vi "PicoScope4000aExampleRapidBlock.vi"() -> ()   [LabVIEW 2016]
uses:
  PicoScope4000aLib/PicoScope4000aAnalogChannelSettings.ctl
panel:
  out "USB 3.0 on non-USB 3.0 port":bool=TRUE
  out "USB powered":bool=TRUE
  in  "Trigger Settings":T1={"Trigger Enabled"=FALSE, "Trigger Source"=enum."Channel A", "Trigger Threshold (Volts/Probe Units)"=0.0, "Trigger Direction"=2, "Trigger Delay (samples)"=0, "Auto Trigger Time (ms)"=0} {"Trigger Direction" items=["Rising"=2, "Falling"=3]}
  in  "Resolution":u32(ring)=1 items=["8-bit", "12-bit", "14-bit"]
  in  "Serial Number":string
  in  "Open using Serial Number":bool
  in  "Channel A Settings":T2={"Enabled"=TRUE, "Coupling"=1, "Range"=6, "Analogue Offset"=0.0, "Bandwidth Limit"=0} {"Bandwidth Limit" items=["Full", "20kHz", "100kHz", "1MHz"]; "Range" items=["10 mV", "20 mV", "50 mV", "100 mV", "200 mV", "500 mV", "1 V", "2 V", "5 V", "10 V", "20 V", "50 V ", "100 V"]; "Coupling" items=["AC", "DC"]}
  in  "Rapid Block Acquisition Settings":T3={"preTriggerSamples"=0, "postTriggerSamples"=1024, "timebase"=10, "Number of Captures"=100}
  out "Capture Complete":bool
  in  "Run":bool
  out "Channel A":i16[][](graph)
  in  "Capture Index":i16 min=0
  in  "stop":bool
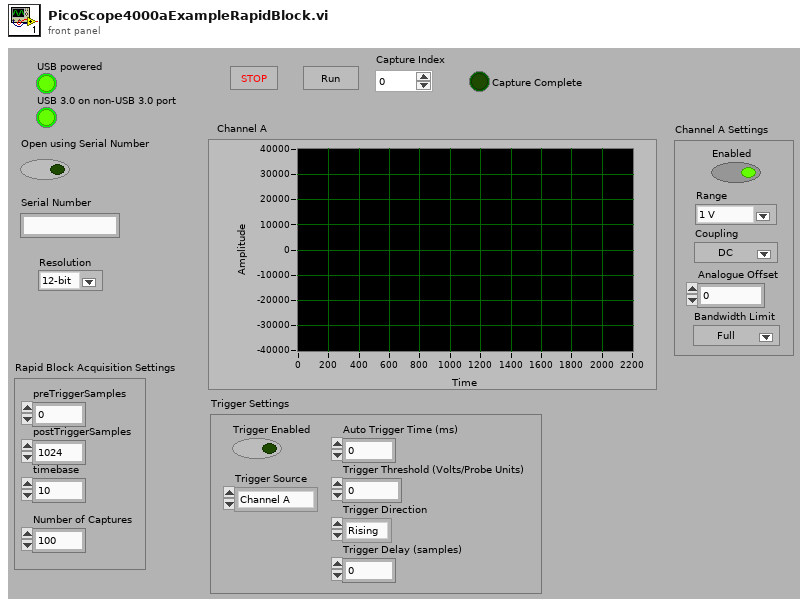
[diagram p1: front panel]
types:
  T1 = cluster{"Trigger Enabled":bool, "Trigger Source":enum16{"Channel A", "Channel B", "Channel C", "Channel D", "Channel E", "Channel F", "Channel G", "Channel H"}, "Trigger Threshold (Volts/Probe Units)":dbl, "Trigger Direction":u16, "Trigger Delay (samples)":u32, "Auto Trigger Time (ms)":i16}
  T2 = typedef "PicoScope4000aAnalogChannelSettings.ctl" = cluster{"Enabled":bool, "Coupling":i16, "Range":u16, "Analogue Offset":sgl, "Bandwidth Limit":u32}
  T3 = cluster{"preTriggerSamples":u32, "postTriggerSamples":u32, "timebase":u32, "Number of Captures":u32}
  T4 = cluster{"Driver Version":string, "USB Version":string, "Hardware":string, "Variant":string, "Batch and Serial":string, "Cal Date":string, "Kernel Version":string, "Digital HW Version":string, "Analogue HW Version":string, "Firmware 1":string, "Firmware 2":string, "Num. channels":i16}
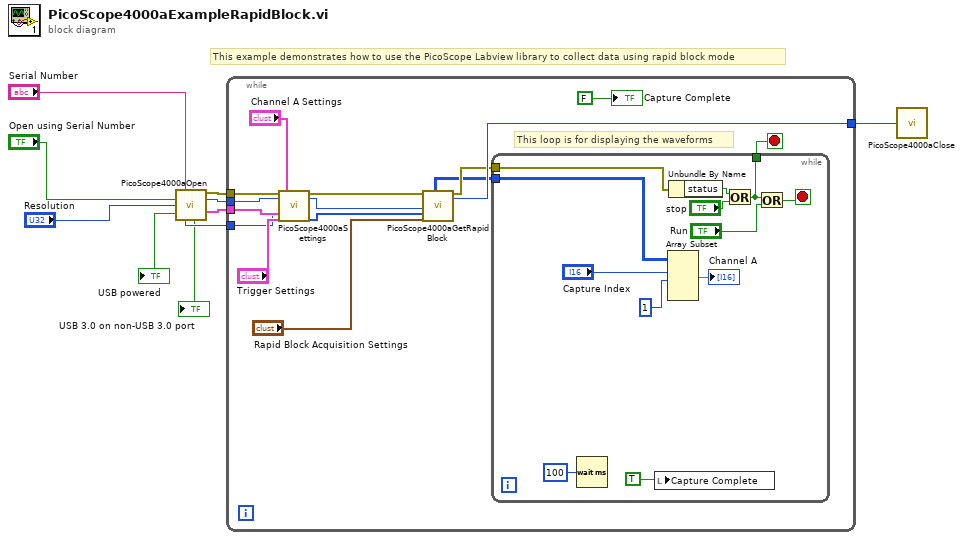
[diagram p0: block diagram]
diagram:
  # "This example demonstrates how to use the PicoScope Labview library to collect data using rapid block mode"
  n1 = call "PicoScope4000aOpen.vi"("Serial Number"="Serial Number", "Use Serial Number"="Open using Serial Number", "Resolution"="Resolution") -> ("error out"=w7:errorcluster, "handle"=w6:i16, "Unit Info"=w5:T4, "Max ADC value"=w3:i16, "USB powered"=→"USB powered":bool, "USB 3.0 on non-USB 3.0 port"=→"USB 3.0 on non-USB 3.0 port":bool)  [unwired: 7 in]
  n2 = while {
    tunnel: [w17] -> w10
    tunnel: w7 -> [w22]
    tunnel: w6 -> [w23]
    tunnel: w5 -> [w13]
    tunnel: w3 -> [w11]
    stop <- w25 stop-if-true
    # "This loop is for displaying the waveforms"
    n3 = call "PicoScope4000aSettings.vi"("error in"=w22, "handle in"=w23, "Max ADC value"=w11, "Trigger Settings"="Trigger Settings", "Channel A Settings"="Channel A Settings", "Unit Info"=w13) -> ("error out"=w19:errorcluster, "handle out"=w18:i16, "Enabled array"=w14:i16[])  [unwired: 11 in]
    n4 = call "PicoScope4000aGetRapidBlock.vi"("error in"=w19, "handle in"=w18, "Enabled array"=w14, "Rapid Block Acquisition Settings"="Rapid Block Acquisition Settings") -> ("Channel A Buffer"=w15:i16[][], "error out"=w16:errorcluster, "handle out"=w17:i16)  [unwired: 6 in, 7 out]
    n5 = while {
      tunnel: [w34] -> w25
      tunnel: w15 -> [w29]
      tunnel: w16 -> [w28]
      stop <- w33 stop-if-true
      n6 = Wait (ms)(milliseconds to wait=u32 100) -> ()  [unwired: 1 out]
      n7 = local write "Capture Complete"(TRUE ("Capture Complete")) -> ()
      n8 = Array Subset(array=w29, index (row)="Capture Index", length (row)=1 ("length")) -> (→"Channel A":i16[][])  [unwired: 2 in]
      n9 = Unbundle By Name(w28) -> ("status"=w27:bool)
      n10 = Or(x=w27, y="stop") -> (x .or. y?=w34:bool)
      n11 = Or(x=w34, y="Run") -> (x .or. y?=w33:bool)
    }
    "Capture Complete" <- FALSE ("Capture Complete")
  }
  n12 = call "PicoScope4000aClose.vi"("handle"=w10) -> ()
